vi "UsrProfiles-Save to Previous Session ini file.vi"(8 "error in":errorcluster) -> ()   [LabVIEW 2020]
uses:
  Typedefs/Save-Load enum.ctl
  Typedefs/Which path.ctl
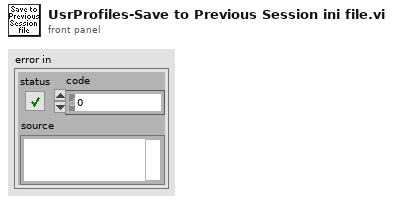
[diagram p1: front panel]
types:
  T1 = typedef "Save-Load enum.ctl" = enum16{"Save to file", "Load from file", "Compare from file", "Save Backup"}
  T2 = typedef "Which path.ctl" = enum16{"Configuration Files", "Calibration Files", "Images", "Setup.ini", "Loaded User profile.ini", "User's-Previous session.ini", "New user profile.ini", "Selected User profile.ini", "User profiles folder", "Power meter scaling.txt", "FOV Cal.ini", "Calibration.ini"}
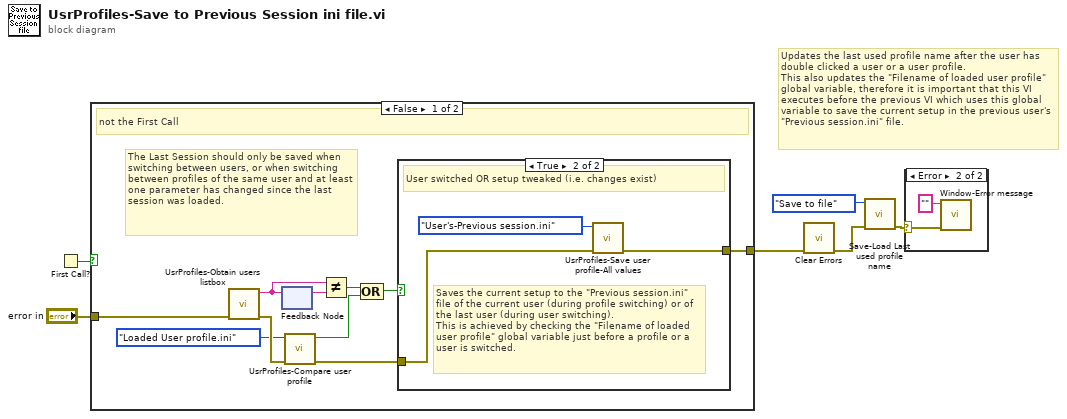
[diagram p0: block diagram]
diagram:
  # "Updates the last used profile name after the user has double clicked a user or a user profile.\nThis also updates the \"Filename of loaded user profile\" global variable, therefore it is important that this VI executes before the previous VI which uses this global variable to save the current setup in the previous user's \"Previous session.ini\" file."
  n1 = First Call?() -> (First Call?: T/F=w1:bool)
  n2 = case shown="False" w1 {
    tunnel: [w16 w21] -> w5
    tunnel: "error in" -> [w7 w21]
    frame False {
      # "The Last Session should only be saved when switching between users, or when switching between profiles of the same user and at least one parameter has changed since the last session was loaded."
      # "not the First Call"
      n3 = call "UsrProfiles-Obtain users listbox.vi"("error in (no error)"=w7) -> ("error out"=w15:errorcluster, "Selected user's name"=w12:string)  [unwired: 7 in, 2 out]
      n4 = feedback #1() -> (w11:string)  [unwired: 1 in]
      n5 = feedback-in #1(w12) -> ()
      n6 = call "UsrProfiles-Compare user profile.vi"("error in"=w15, "Which profile?"=Which_path."Loaded User profile.ini" ("Which file?")) -> ("error out"=w8:errorcluster, "Changes exist"=w14:bool)  [unwired: 8 in]
      n7 = Not Equal?(x=w12, y=w11) -> (x != y?=w13:bool)
      n8 = Compound Arithmetic op=OR(w13, w14) -> (w9:bool)
      n9 = case shown="True" w9 {
        tunnel: [w17 w20] -> w16
        tunnel: w8 -> [w17 w18]
        frame False {
          # "Do not save to the 'Previous Session' profile."
        }
        frame True {
          # "Saves the current setup to the \"Previous session.ini\" file of the current user (during profile switching) or of the last user (during user switching).\nThis is achieved by checking the \"Filename of loaded user profile\" global variable just before a profile or a user is switched."
          # "User switched OR setup tweaked (i.e. changes exist)"
          n10 = call "UsrProfiles-Save user profile-All values.vi"("error in"=w18, "Which file? (User profile.ini)"=Which_path."User's-Previous session.ini" ("Which file?")) -> ("error out"=w20:errorcluster)  [unwired: 9 in]
        }
      }
    }
    frame True {
      # "First Call"
    }
  }
  n11 = call <vilib>:"Clear Errors.vi"("error in (no error)"=w5) -> ("error out"=w6:errorcluster)  [unwired: 5 in, 1 out]
  n12 = call "Save-Load Last used profile name.vi"("error in"=w6, "Function"=Save-Load_enum."Save to file") -> ("error out"=w3:errorcluster)  [unwired: 7 in, 2 out]
  n13 = case shown="Error" w3 {
    selector: w3 -> [_ w23]
    frame No Error {
    }
    frame Error {
      n14 = call "Window-Error message.vi"("error in (no error)"=w23, "Message"="") -> ()  [unwired: 9 in, 1 out]
    }
  }
